vi "Trigger.vi"(8 "error in (no error)":errorcluster, 9 "Parameter":variant, 10 "Function":string, 11 "input in":refnum<class "input.lvclass">) -> (0 "error out":errorcluster, 3 "input out":refnum<class "input.lvclass">)   [LabVIEW 2015, in "input.lvclass"]
uses:
  input.lvclass
  input.lvclass/input.ctl
  <vilib>/addons/lv-msgpack/MsgPack Serializer/MsgPackSerializer.lvclass
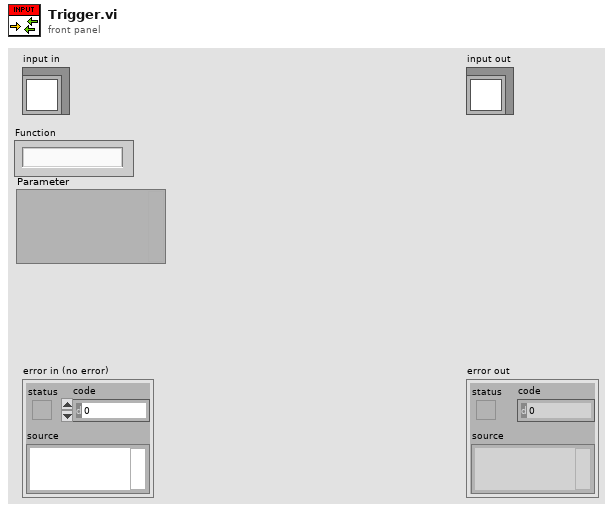
[diagram p1: front panel]
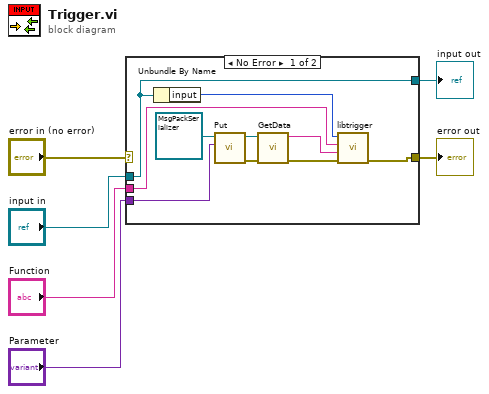
[diagram p0: block diagram]
diagram:
  n1 = case shown="No Error" "error in (no error)" {
    selector: "error in (no error)" -> [_ w18]
    tunnel: [w11 w18] -> w5
    tunnel: [w8 w17] -> w3
    tunnel: "input in" -> [w8 w17]
    tunnel: "Parameter" -> [w13 _]
    tunnel: "Function" -> [w10 _]
    frame No Error {
      n2 = Unbundle By Name(w8) -> ("input"=w7:i32)
      n3 = call <vilib>:"Put.vi"("Data"=w13, "MsgPackSerializer in"=refnum<class "MsgPackSerializer.lvclass"> refnum) -> ("error out"=w16:errorcluster, "MsgPackSerializer out"=w15:refnum<class "MsgPackSerializer.lvclass">)  [unwired: 8 in]
      n4 = call <vilib>:"GetData.vi"("error in (no error)"=w16, "MsgPackSerializer in"=w15) -> ("error out"=w12:errorcluster, "Data"=w9:string)  [unwired: 8 in]
      n5 = call "libtrigger.vi"("error in (no error)"=w12, "Parameter"=w9, "Function"=w10, "input"=w7) -> ("error out"=w11:errorcluster)  [unwired: 7 in]
    }
    frame Error {
    }
  }
  "error out" <- w5
  "input out" <- w3
